vi "RDS Child Launch and Subscribe.vi"(8 "error in (no error)":errorcluster, 10 "RDS Child in":refnum<class "RDS Parent Actor.lvclass">, 11 "Caller Actor in":refnum<class "Actor.lvclass">) -> (0 "error out":errorcluster, 2 "Nested Actor's Enqueuer":refnum<class "Message Enqueuer.lvclass">, 3 "Caller Actor Out":refnum<class "Actor.lvclass">)   [LabVIEW 2015, in "RDS Abstracts.lvlib" / "RDS Parent Actor.lvlib" / "RDS Parent Actor.lvclass"]
doc: "This VI tidy's up the launching of an RDS child actor. The extra thing it is doing is creating the RDS message subscription, storing the router's enqueur as private data and sending the subscription request message to the router."
uses:
  RDS Parent Actor.lvclass
  <vilib>/ActorFramework/Actor/Actor.lvclass
  <vilib>/ActorFramework/Message Enqueuer/Message Enqueuer.lvclass
  RDS Root Actor/RDS Root Actor/RDS Root Actor.lvclass
  RDS Root Actor/RDS Root Actor/RDS Root Actor.lvclass/RDS Root Actor.ctl
  RDS Parent Actor.lvclass/RDS Parent Actor.ctl
  RDS Router Actor/RSD Subscription Class/RDS Router Subscription.lvclass
  RDS Router Actor/RDS Router Actor Messages/RDS Router Subscribe Msg/RDS Router Subscribe Msg.lvclass
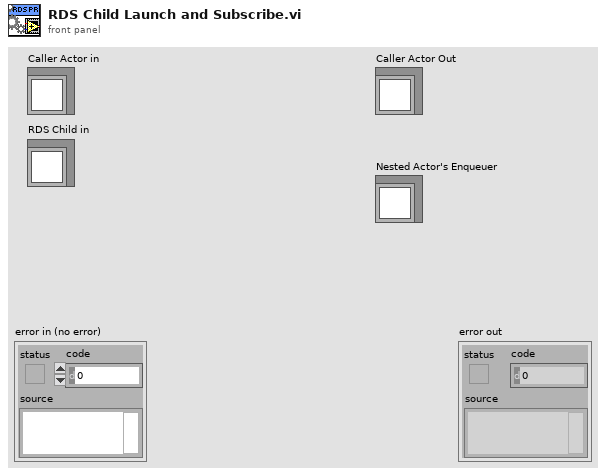
[diagram p1: front panel]
types:
  T1 = typedef "RDS Child Messages.lvlib/RDS Message ID.ctl" = enum16{"RDS Hello World", "String Message", "AIP_Status", "AIP_Command", "GPS_Data", "MCB_Command", "MCB_Status", "Compass_Data", "Depth_Data", "Battery_Data", "Contoller_State", "Set_Mag_Dev", "BTB_Shutdown", "State_Sample_Request", "State_Sample", "PID_Gains_Set", "Helm_Limiter_Set", "Helm_Heading_Command", "Helm_Steering_Command", "Helm_Status", "Controller_Message", "AIP_Set_Min_Depth", "Mission_Controller_State", "Mission_Upload", "Mission_Set_Op_and_Run", "Mission_Settings_Set"}
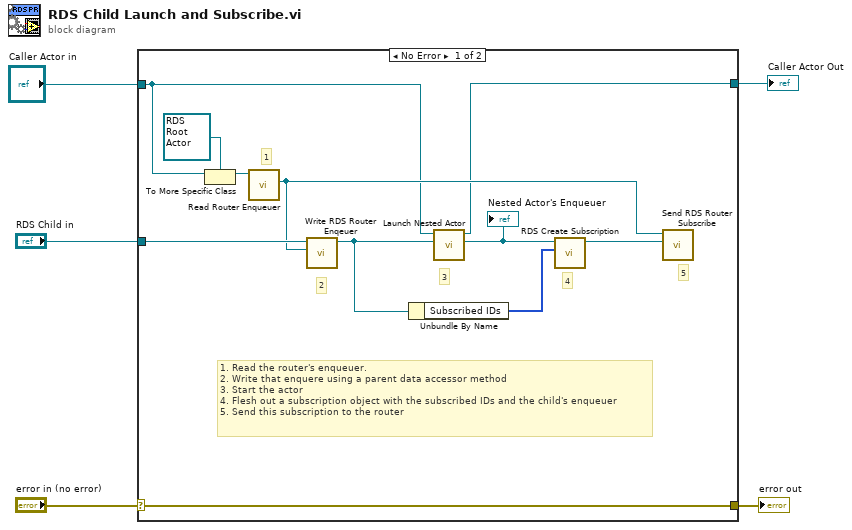
[diagram p0: block diagram]
diagram:
  n1 = case shown="No Error" "error in (no error)" {
    selector: "error in (no error)" -> [w16 w18]
    tunnel: [w16 w18] -> w4
    tunnel: [w6 w17] -> w2
    tunnel: "RDS Child in" -> [w15 _]
    tunnel: "Caller Actor in" -> [w7 w17]
    frame No Error {
      # "5"
      # "4"
      # "3"
      # "2"
      # "1. Read the router's enqueuer. \n2. Write that enquere using a parent data accessor method\n3. Start the actor\n4. Flesh out a subscription object with the subscribed IDs and the child's enqueuer\n5. Send this subscription to the router"
      # "1"
      n2 = To More Specific Class(target class=refnum<class "RDS Root Actor.lvclass"> refnum ("RDS Root Actor.lvlib:RDS Root Actor.lvclass"), reference=w7) -> (specific class reference=w8:refnum<class "RDS Root Actor.lvclass">)  [unwired: 1 in, 1 out]
      n3 = call "Read Router Enqueuer.vi"("RDS Root Actor in"=w8) -> ("Actor Framework:Message Enqueuer"=w11:refnum<class "Message Enqueuer.lvclass">)  [unwired: 8 in, 2 out]
      n4 = call "Write RDS Router Enqeuer.vi"("RDS Router Enqueuer"=w11, "RDS Child Actor in"=w15) -> ("RDS Child Actor out"=w13:refnum<class "RDS Parent Actor.lvclass">)  [unwired: 8 in, 1 out]
      n5 = Unbundle By Name(w13) -> ("Subscribed IDs"=w12:T1[])
      n6 = call <vilib>:"Launch Nested Actor.vi"("Nested Actor"=w13, "Caller Actor in"=w7) -> ("Nested Actor's Enqueuer"=w10:refnum<class "Message Enqueuer.lvclass">, "Caller Actor out"=w6:refnum<class "Actor.lvclass">)  [unwired: 7 in, 1 out]
      "Nested Actor's Enqueuer" <- w10
      n7 = call "RDS Create Subscription.vi"("Subscribed IDs"=w12, "RDS Child Enqueuer"=w10) -> ("RDS Router Subscription out"=w14:refnum<class "RDS Router Subscription.lvclass">)  [unwired: 8 in, 1 out]
      n8 = call "Send RDS Router Subscribe.vi"("RDS Router Subscription"=w14, "Message Enqueuer in"=w11) -> ()  [unwired: 8 in, 2 out]
    }
    frame Error {
    }
  }
  "error out" <- w4
  "Caller Actor Out" <- w2
